vi "onPrevious.vi"(8 "error in (no error)":errorcluster, 11 "LockedState in":refnum<class "LockedState.lvclass">) -> (0 "error out":errorcluster, 2 "String":string, 3 "LockedState out":refnum<class "LockedState.lvclass">)   [LabVIEW 2016, in "LockedState.lvclass"]
uses:
  LockedState.lvclass
  State Class/State.lvclass
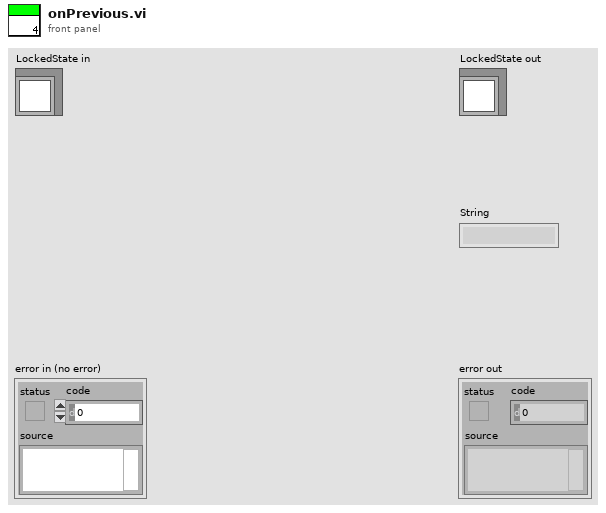
[diagram p1: front panel]
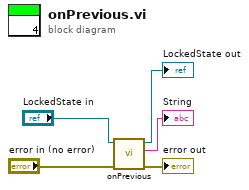
[diagram p0: block diagram]
diagram:
  n1 = call-parent "onPrevious.vi"("error in (no error)"="error in (no error)", "State in"="LockedState in") -> ("error out"=→"error out":errorcluster, "String"=→"String":string, "State out"=→"LockedState out":refnum<class "LockedState.lvclass">)  [unwired: 7 in]
